vi "Flock_Shared_Intialize Queue.vi"(8 "error in (no error)":errorcluster, 11 "Enum":T1) -> (0 "error out":errorcluster, 3 "Process Name":T1)   [LabVIEW 2013, in "Flock_Shared_Messaging.lvlib" / "Flock_Shared_LocalProcessMessaging.lvlib"]
uses:
  Flock_Shared_LocalProcessMessaging.lvlib
  FGV_Action.ctl
  Flock_Shared_Messaging.lvlib
  ProcessList.ctl
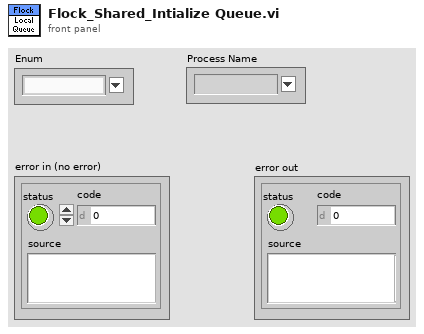
[diagram p1: front panel]
types:
  T1 = typedef "Flock_Shared_Messaging.lvlib/ProcessList.ctl" = string
  T2 = typedef "FGV_Action.ctl" = enum16{"Initalize Central", "Initialize Local", "Get", "Delete Local"}
  T3 = typedef "AMC.lvlib/Message Queue.ctl" = refnum<queue>
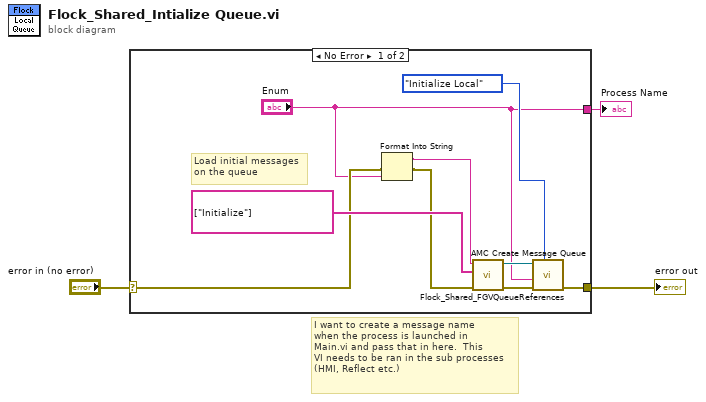
[diagram p0: block diagram]
diagram:
  # "I want to create a message name\nwhen the process is launched in \nMain.vi and pass that in here.  This\nVI needs to be ran in the sub processes\n(HMI, Reflect etc.)"
  n1 = case shown="No Error" "error in (no error)" {
    selector: "error in (no error)" -> [w7 w13]
    tunnel: [w9 w13] -> w3
    tunnel: ["Enum" _] -> w1
    frame No Error {
      # "Load initial messages\non the queue"
      n2 = Format Into String(error in=w7, "Enum") -> (resulting string=w5:string, error out=w6:errorcluster)  [unwired: 2 in]
      n3 = call <vilib>:"AMC Create Message Queue.vi"("error in (no error)"=w6, "Initial Message Names"=string[] ["Initialize"], "Message Queue Name"=w5) -> ("error out"=w8:errorcluster, "Message Queue out"=w10:T3)  [unwired: 1 in, 6 out]
      n4 = call "Flock_Shared_FGVQueueReferences.vi"("Action"=FGV_Action."Initialize Local", "error in (no error)"=w8, "Queue Name"="Enum", "Local Queue in"=w10) -> ("error out"=w9:errorcluster)  [unwired: 5 in, 2 out]
    }
    frame Error {
    }
  }
  "error out" <- w3
  "Process Name" <- w1
